vi "TestU8ToFXP.vi"(1 "string":string) -> (0 "Output":fxp<+/-,24,8>[](array[numeric]))   [LabVIEW 2018]
panel:
  out "Input":u8[](array[numeric])
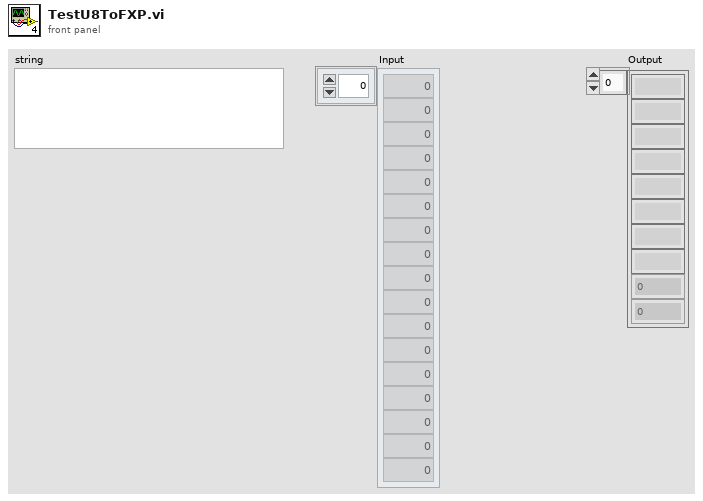
[diagram p1: front panel]
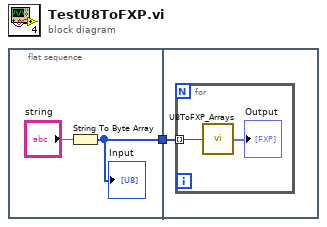
[diagram p0: block diagram]
diagram:
  n1 = flat-sequence {
    tunnel: [w2] -> w1
    tunnel: w1 -> [w4]
    frame #0 {
      n2 = String To Byte Array(string="string") -> (unsigned byte array=w2:u8[])
      "Input" <- w2
    }
    frame #1 {
      n3 = for {
        tunnel: w4 -> [w5] mode=indexing
        n4 = call "U8ToFXP_Arrays.vi"("Input"=w5) -> ("Array"=→"Output":fxp<+/-,24,8>[])
      }
    }
  }
